vi "module-11-analog-position-ctrl.vi"() -> ()   [LabVIEW 2019]
uses:
  Secret_Control_Library_Protected/CtrlTrain_Pos_ctrl_TuningParameters.ctl
  <vilib>/addons/control/pid/pid.llb/PID Lead-Lag (DBL).vi
  <vilib>/addons/control/pid/NI_PID_pid.lvlib
  Secret_Control_Library_Protected/Secret_Control_Library_Protected.lvlib
panel:
  in  "Tab Control":T1(tab)
  in  "Desired Position":dbl(slide) min=0.0 max=90.0 scale=0.0..90.0
  in  "Auto - Set Position To 0 / Manual - Lower":bool
  in  "Auto - Set Position to 90 / Manual - Raise":bool
  in  "Set Position to Desired\n(Select to activate position)":bool
  out "Selected Setpoint \n(In Manual \ntracks Position)":dbl
  out "Current Position 2":dbl format="%.2f"
  out "Motor Demand":dbl format="%#.2f"
  out "Position Error":dbl format="%#3.2f"
  out "SP, PV, CO Chart":T2(graph)
  out "Current Position":dbl(knob) scale=-10.0..100.0
  in  "Auto / Manual":bool=TRUE
  in  "MinLimitSwitch":bool
  in  "MaxLimitSwitch":bool
  out "In Position":bool
  in  "TuningParameters":T3={"MaxOutput"=1.0, "MinOutput"=0.25, "PositionErrThreshold"=6.0, "PositionErrDeadband"=0.5, "ReverseOutput"=FALSE, "PositionMax"=89.0, "PositionMin"=1.0, "WithinDBCount"=5} {"WithinDBCount" min=1}
  out "Current-Setpoint":dbl
  out "Current-Position":dbl
  out "Manual-Lower":bool
  out "Manual-Raise":bool
  out "Motor-Demand":dbl
  # "Example of Closed Loop Position Control Using a Motor\n(Simple Example 002)"
  # "This example adds a \"Manual\" mode so that the arm\ncan still be moved if the position indication fails.\nThis example also adds failsafe min and max positions\nand optional inputs from limit switches to stop the motor \nfrom traveling too far."
  # "This value shows the error between the current position\nand the desired position."
  # "This value shows the current position.  This is measured by an encoder, a potentiometer, or some other sensor.  This is called the \"Process Variable\","
  # "Press one of the buttons to set the desired \nposition.  This \"target\" value is called\nthe \"Set Point\".  In \"Manual\" mode hold the 0 or 90 button\ndown to manually run the motor."
  # "This value shows the current motor output demand.  This\ncould also be a motor speed demand and another closed\nloop controller would control the motor speed.  In this simple\nexample this value is used to drive the simulated motor directly.\nThis motor demand is called the \"Control Output\"."
  # "The action caused by the motor causes the position to change."
  # "Toggle these switches to simulate a limit switch input."
  # "These are the tuning parameters for the Position Control VI"
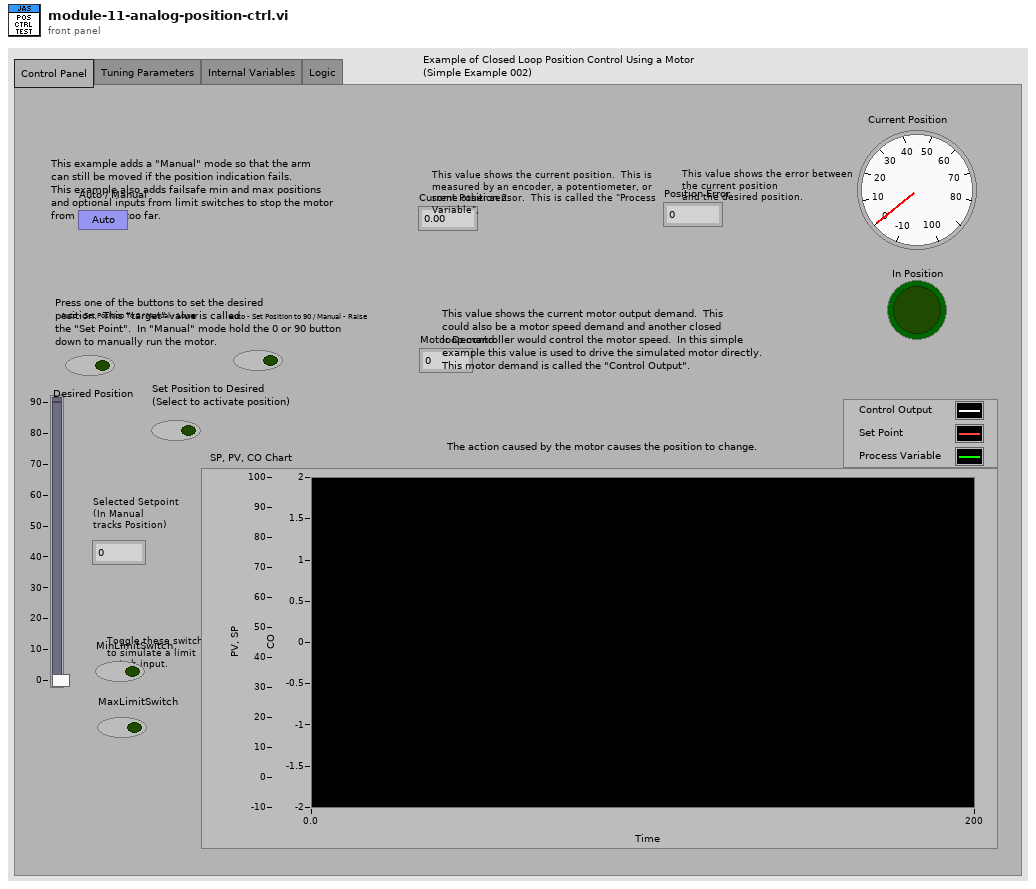
[diagram p1: front panel]
types:
  T1 = enum32{"Control Panel", "Tuning Parameters", "Internal Variables", "Logic"}
  T2 = cluster{"MotorDemand":dbl, "CurrentSetpoint":dbl, "CurrentPosition":dbl}
  T3 = typedef "Secret_Control_Library_Protected.lvlib/CtrlTrain_Pos_ctrl_TuningParameters.ctl" = cluster{"MaxOutput":dbl, "MinOutput":dbl, "PositionErrThreshold":dbl, "PositionErrDeadband":dbl, "ReverseOutput":bool, "PositionMax":dbl, "PositionMin":dbl, "WithinDBCount":i32}
  T4 = cluster{"gain":dbl, "lag time":dbl, "lead time":dbl}
  T5 = cluster{"Motor-Demand":dbl, "Current-Setpoint":dbl, "Current-Position":dbl}
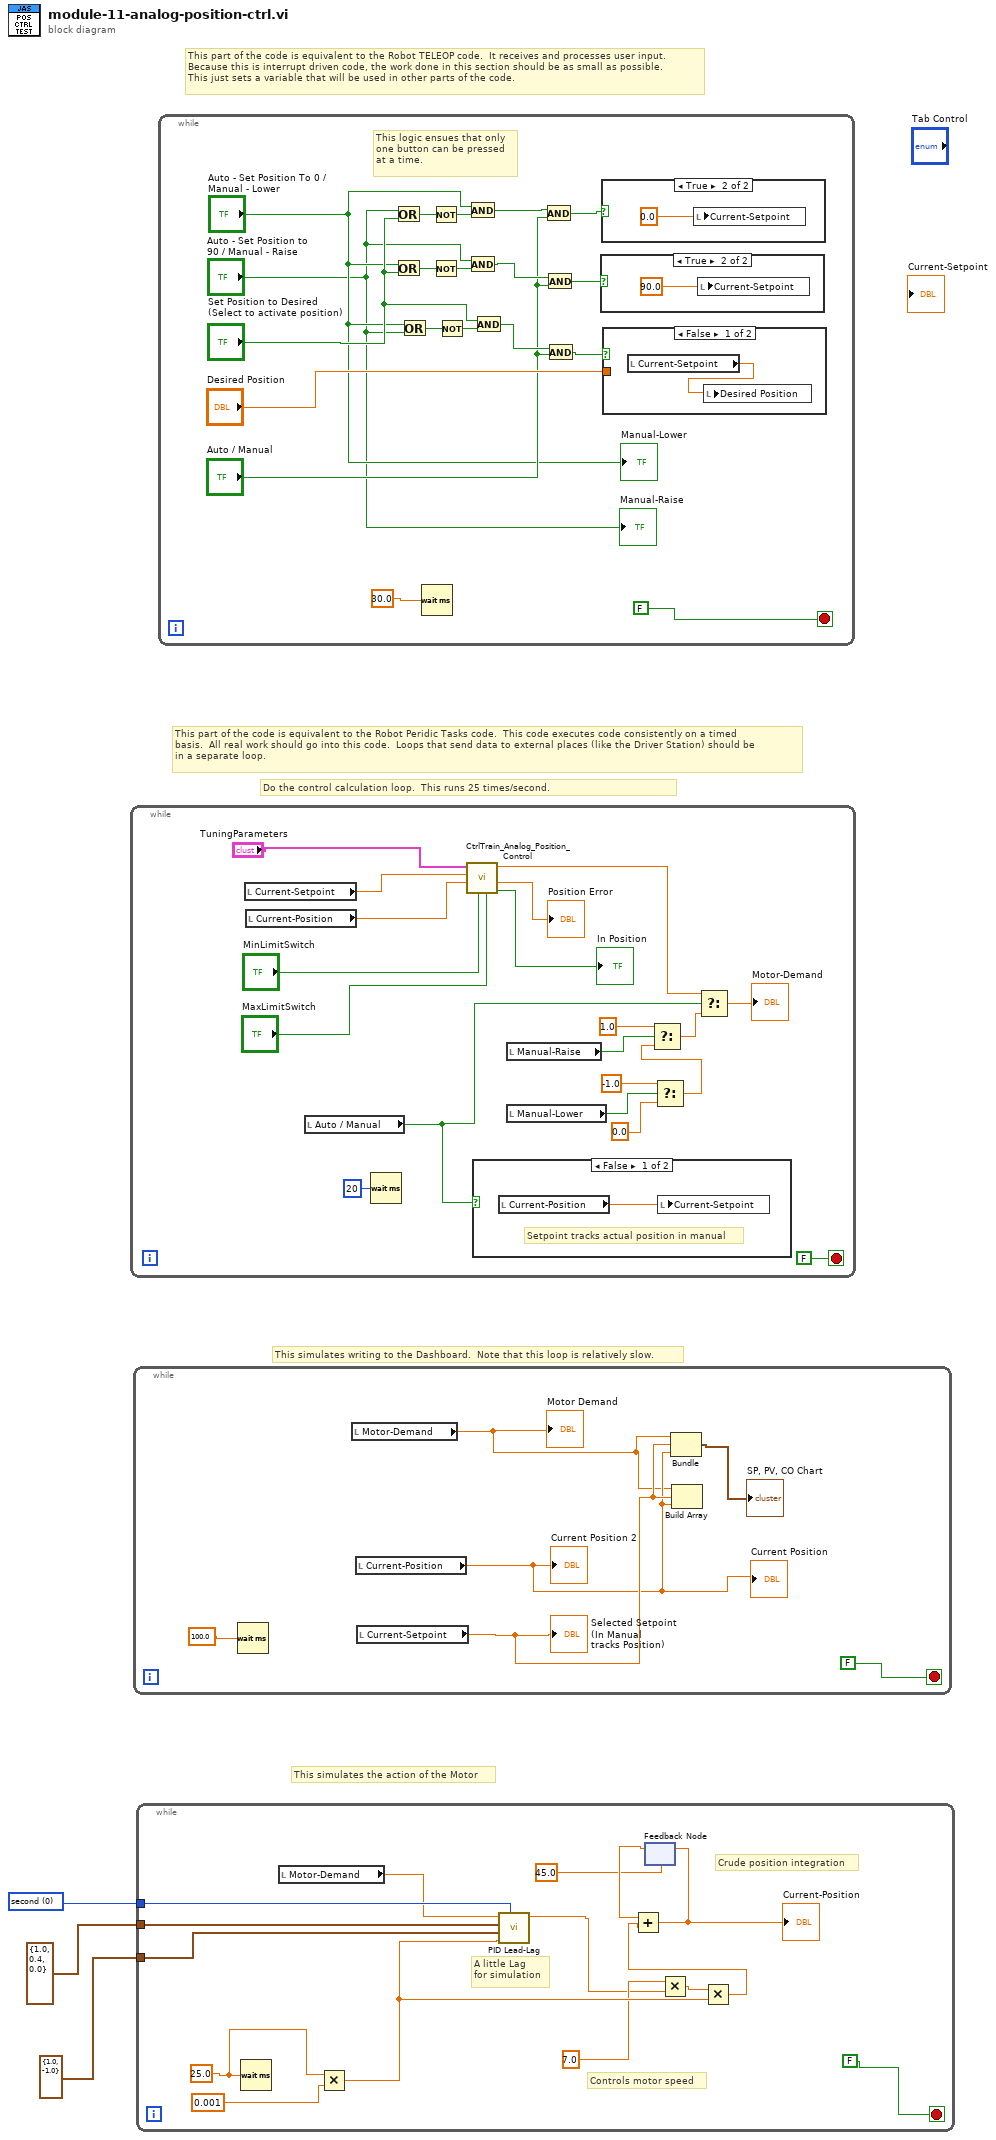
[diagram p0: block diagram]
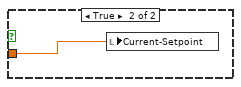
[diagram p3: hidden frame]
diagram:
  w3 = u16 0 items=["second", "minute"] ("time unit")
  # "This simulates the action of the Motor"
  # "This simulates writing to the Dashboard.  Note that this loop is relatively slow."
  # "Do the control calculation loop.  This runs 25 times/second."
  # "This part of the code is equivalent to the Robot Peridic Tasks code.  This code executes code consistently on a timed\nbasis.  All real work should go into this code.  Loops that send data to external places (like the Driver Station) should be \nin a separate loop."
  # "This part of the code is equivalent to the Robot TELEOP code.  It receives and processes user input.\nBecause this is interrupt driven code, the work done in this section should be as small as possible.\nThis just sets a variable that will be used in other parts of the code."
  n1 = while {
    stop <- FALSE stop-if-true
    n2 = local read "Current-Setpoint"() -> (w10:dbl)
    n3 = local read "Current-Position"() -> (w9:dbl)
    n4 = local read "Auto / Manual"() -> (w17:bool)
    n5 = Wait (ms)(milliseconds to wait=u32 20) -> ()  [unwired: 1 out]
    n6 = call "CtrlTrain_Analog_Position_Control.vi"("PositionMax"="MaxLimitSwitch", "PositionMin"="MinLimitSwitch", "CurrentPosition"=w9, "TargetPosition"=w10, "Pos_Ctrl_TuningParameters"="TuningParameters") -> ("OnTarget"=→"In Position":bool, "PositionError"=→"Position Error":dbl, "Output"=w5:dbl)  [unwired: 4 in]
    n7 = case shown="False" w17 {
      frame False {
        # "Setpoint tracks actual position in manual"
        n8 = local read "Current-Position"() -> (w23:dbl)
        n9 = local write "Current-Setpoint"(w23) -> ()
      }
      frame True {
      }
    }
    n10 = local read "Manual-Raise"() -> (w16:bool)
    n11 = local read "Manual-Lower"() -> (w15:bool)
    n12 = Select(t=-1.0, s=w15, f=0.0) -> (s? t:f=w19:dbl)
    n13 = Select(t=1.0, s=w16, f=w19) -> (s? t:f=w18:dbl)
    n14 = Select(t=w5, s=w17, f=w18) -> (s? t:f=→"Motor-Demand":dbl)
  }
  n15 = while {
    stop <- FALSE stop-if-true
    n16 = Wait (ms)(milliseconds to wait=100.0) -> ()  [unwired: 1 out]
    n17 = local read "Motor-Demand"() -> (w24:dbl)
    "Motor Demand" <- w24
    n18 = local read "Current-Position"() -> (w25:dbl)
    "Current Position 2" <- w25
    "Current Position" <- w25
    n19 = local read "Current-Setpoint"() -> (w26:dbl)
    "Selected Setpoint \n(In Manual \ntracks Position)" <- w26
    n20 = Bundle("Motor-Demand"=w24, "Current-Setpoint"=w26, "Current-Position"=w25) -> (→"SP, PV, CO Chart":T5)  [unwired: 1 in]
    n21 = Build Array(w24, w26, w25) -> ()  [unwired: 1 out]
  }
  n22 = while {
    tunnel: w3 -> [w44]
    tunnel: T4 {"gain"=1.0, "lag time"=0.4, "lead time"=0.0} ("tuning parameters") -> [w43]
    tunnel: cluster{"output high":dbl, "output low":dbl} {"output high"=1.0, "output low"=-1.0} ("output range") -> [w41]
    stop <- FALSE stop-if-true
    w33 = 25.0
    # "Controls motor speed"
    # "Crude position integration"
    # "A little Lag\nfor simulation"
    n23 = Wait (ms)(milliseconds to wait=w33) -> ()  [unwired: 1 out]
    n24 = local read "Motor-Demand"() -> (w30:dbl)
    n25 = Multiply(x=w33, y=0.001) -> (x*y=w40:dbl)
    n26 = call-poly <vilib>:"PID Lead-Lag.vi"("time unit"=w44, "dt (s)"=w40, "output range"=w41, "tuning parameters"=w43, "input"=w30) -> ("output"=w32:dbl)  [unwired: 3 in, 1 out]
    n27 = feedback #1(45.0) -> (w38:dbl)
    n28 = Multiply(x=7.0, y=w32) -> (x*y=w39:dbl)
    n29 = Multiply(x=w39, y=w40) -> (x*y=w36:dbl)
    n30 = Add(x=w38, y=w36) -> (x+y=w31:dbl)
    "Current-Position" <- w31
    n31 = feedback-in #1(w31) -> ()
  }
  n32 = while {
    stop <- FALSE stop-if-true
    # "This logic ensues that only\none button can be pressed\nat a time."
    n33 = Or(x="Auto - Set Position to 90 / Manual - Raise", y="Set Position to Desired\n(Select to activate position)") -> (x .or. y?=w63:bool)
    n34 = Or(x="Auto - Set Position To 0 / Manual - Lower", y="Set Position to Desired\n(Select to activate position)") -> (x .or. y?=w61:bool)
    n35 = Or(x="Auto - Set Position To 0 / Manual - Lower", y="Auto - Set Position to 90 / Manual - Raise") -> (x .or. y?=w59:bool)
    n36 = Wait (ms)(milliseconds to wait=30.0) -> ()  [unwired: 1 out]
    n37 = Not(x=w63) -> (.not. x?=w62:bool)
    n38 = Not(x=w61) -> (.not. x?=w60:bool)
    n39 = Not(x=w59) -> (.not. x?=w58:bool)
    n40 = And(x="Auto - Set Position To 0 / Manual - Lower", y=w62) -> (x .and. y?=w53:bool)
    n41 = And(x="Auto - Set Position to 90 / Manual - Raise", y=w60) -> (x .and. y?=w49:bool)
    n42 = And(x="Set Position to Desired\n(Select to activate position)", y=w58) -> (x .and. y?=w48:bool)
    n43 = And(x=w53, y="Auto / Manual") -> (x .and. y?=w52:bool)
    n44 = And(x=w49, y="Auto / Manual") -> (x .and. y?=w51:bool)
    n45 = And(x=w48, y="Auto / Manual") -> (x .and. y?=w50:bool)
    n46 = case shown="True" w51 {
      frame False {
      }
      frame True {
        n47 = local write "Current-Setpoint"(90.0) -> ()
      }
    }
    n48 = case shown="True" w52 {
      frame False {
      }
      frame True {
        n49 = local write "Current-Setpoint"(0.0) -> ()
      }
    }
    n50 = case shown="False" w50 {
      tunnel: "Desired Position" -> [_ w65]
      frame False {
        n51 = local read "Current-Setpoint"() -> (w64:dbl)
        n52 = local write "Desired Position"(w64) -> ()
      }
      frame True {
        n53 = local write "Current-Setpoint"(w65) -> ()
      }
    }
    "Manual-Raise" <- "Auto - Set Position to 90 / Manual - Raise"
    "Manual-Lower" <- "Auto - Set Position To 0 / Manual - Lower"
  }
